vi "Test Program Data Array.vi"(8 "error in (no error)":errorcluster, 11 "Data Cluster in":T1) -> (0 "error out":errorcluster, 2 "Task D-O Channels":string[][](array[string]), 3 "Data Cluster out":T1)   [LabVIEW 2018, in "DAQ.lvlib"]
uses:
  DAQ.lvlib
  <resource>/objmgr/daqmx.rc
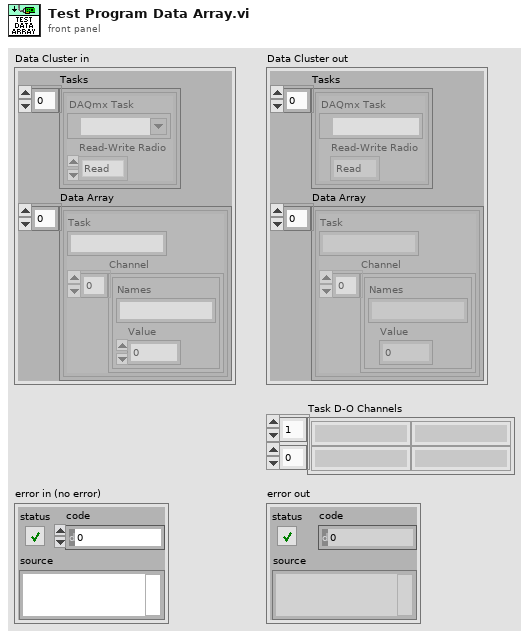
[diagram p1: front panel]
types:
  T1 = cluster{"Tasks":cluster{"DAQmx Task":refnum<k21>, "Read-Write Radio":enum32{"Read", "Write"}}[], "Data Array":cluster{"Task":string, "Channel":cluster{"Names":string, "Value":dbl}[]}[]}
  T2 = cluster{"DAQmx Task":refnum<k21>, "Read-Write Radio":enum32{"Read", "Write"}}[]
  T3 = cluster{"Task":string, "Channel":cluster{"Names":string, "Value":dbl}[]}[]
  T4 = cluster{"Task":string, "Channel":cluster{"Names":string, "Value":dbl}[]}
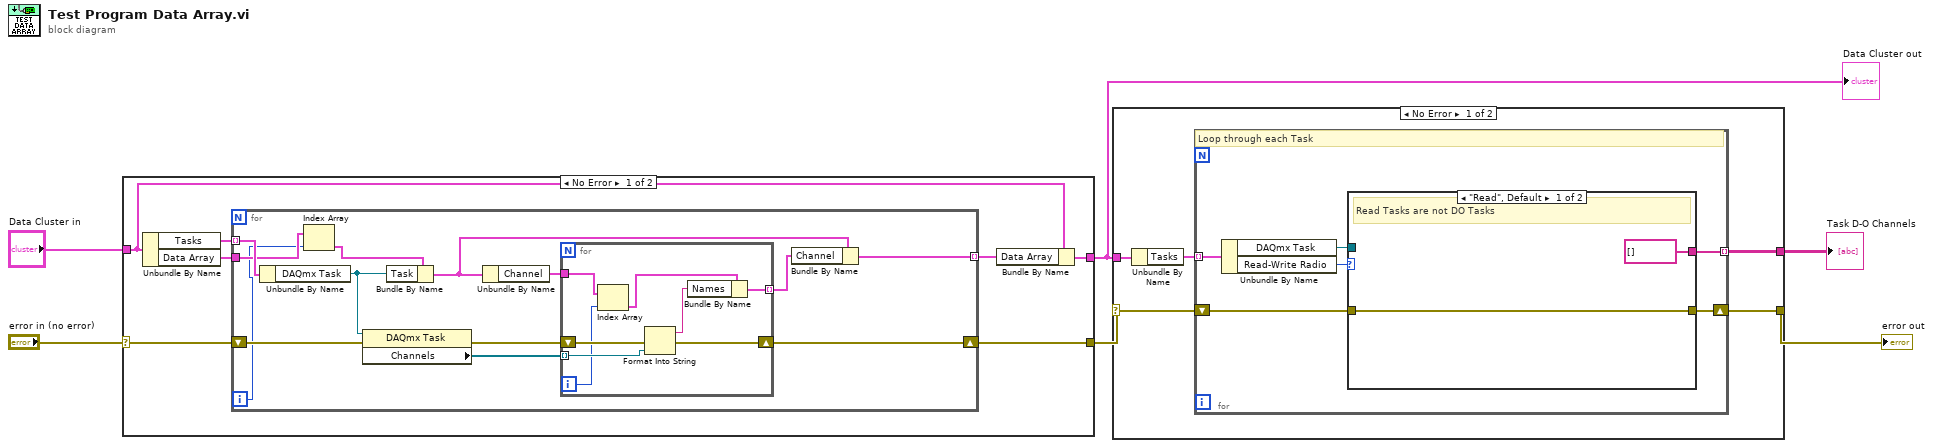
[diagram p0: block diagram]
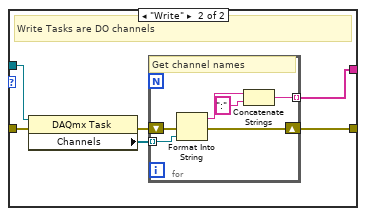
[diagram p2: hidden frame]
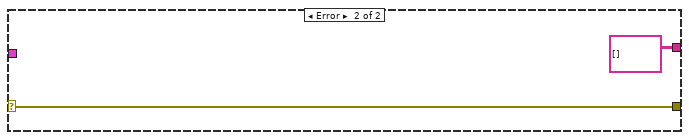
[diagram p3: hidden frame]
diagram:
  n1 = case shown="No Error" "error in (no error)" {
    selector: "error in (no error)" -> [w12 w36]
    tunnel: "Data Cluster in" -> [w9 w35]
    tunnel: [w11 w36] -> w6
    tunnel: [w7 w35] -> w5
    frame No Error {
      n2 = Unbundle By Name(w9) -> ("Tasks"=w13:T2, "Data Array"=w10:T3)
      n3 = for {
        tunnel: w13 -> [w26] mode=indexing
        shift-right: [w23] -> w11
        shift-left: w12 -> [w25]
        tunnel: w10 -> [w17]
        tunnel: [w18] -> w8 mode=indexing
        i -> [w16]
        n4 = Unbundle By Name(w26) -> ("DAQmx Task"=w21:refnum<k21>)
        n5 = Index Array(array=w17, index=w16) -> (element=w15:T4)
        n6 = property class="DAQmx Task"(reference=w21, error in=w25) -> (error out=w22:errorcluster, "Channels"=w24:refnum<k21>[])  [unwired: 1 out]
        n7 = Bundle By Name(cluster=w15, "Task"=w21) -> (w14:T4)
        n8 = Unbundle By Name(w14) -> ("Channel"=w20:cluster{"Names":string, "Value":dbl}[])
        n9 = for {
          tunnel: w24 -> [w33] mode=indexing
          shift-right: [w34] -> w23
          shift-left: w22 -> [w32]
          tunnel: w20 -> [w28]
          tunnel: [w30] -> w19 mode=indexing
          i -> [w29]
          n10 = Index Array(array=w28, index=w29) -> (element=w27:cluster{"Names":string, "Value":dbl})
          n11 = Format Into String(error in=w32, w33) -> (resulting string=w31:string, error out=w34:errorcluster)  [unwired: 2 in]
          n12 = Bundle By Name(cluster=w27, "Names"=w31) -> (w30:cluster{"Names":string, "Value":dbl})
        }
        n13 = Bundle By Name(cluster=w14, "Channel"=w19) -> (w18:T4)
      }
      n14 = Bundle By Name(cluster=w9, "Data Array"=w8) -> (w7:T1)
    }
    frame Error {
    }
  }
  "Data Cluster out" <- w5
  n15 = case shown="No Error" w6 {
    selector: w6 -> [w38 w63]
    tunnel: w5 -> [w40 _]
    tunnel: [w39 w63] -> w2
    tunnel: [w37 string[][] []] -> w3
    frame No Error {
      n16 = Unbundle By Name(w40) -> ("Tasks"=w41:T2)
      n17 = for {
        tunnel: w41 -> [w47] mode=indexing
        shift-right: [w44] -> w39
        shift-left: w38 -> [w42]
        tunnel: [w45] -> w37 mode=indexing
        # "Loop through each Task"
        n18 = Unbundle By Name(w47) -> ("DAQmx Task"=w43:refnum<k21>, "Read-Write Radio"=w46:enum32{"Read", "Write"})
        n19 = case shown="\"Read\", Default" w46 {
          tunnel: [string[] [] w50] -> w45
          tunnel: [w49 w55] -> w44
          tunnel: w43 -> [_ w54]
          tunnel: w42 -> [w49 w53]
          frame "Read", Default {
            # "Read Tasks are not DO Tasks"
          }
          frame "Write" {
            # "Write Tasks are DO channels"
            n20 = property class="DAQmx Task"(reference=w54, error in=w53) -> (error out=w52:errorcluster, "Channels"=w51:refnum<k21>[])  [unwired: 1 out]
            n21 = for {
              tunnel: w51 -> [w61] mode=indexing
              shift-right: [w59] -> w55
              shift-left: w52 -> [w60]
              tunnel: [w56] -> w50 mode=indexing
              # "Get channel names"
              n22 = Format Into String(error in=w60, w61) -> (resulting string=w58:string, error out=w59:errorcluster)  [unwired: 2 in]
              n23 = Concatenate Strings(w58, ":" ("string")) -> (w56:string)
            }
          }
        }
      }
    }
    frame Error {
    }
  }
  "error out" <- w2
  "Task D-O Channels" <- w3
